vi "SetVIRef.vi"(8 "error in (no error)":errorcluster, 10 "VI Refnum":refnum<vi>, 11 "WindowFrame in":refnum<class "WindowFrame.lvclass">) -> (0 "error out":errorcluster, 3 "WindowFrame out":refnum<class "WindowFrame.lvclass">)   [LabVIEW 2021, in "WindowFrame.lvlib" / "WindowFrame.lvclass"]
uses:
  WindowFrame.lvclass
  C:/GitHub/ClassUtilities/src/ClassByRef/ClassByRef.lvclass
  ClassUtilities/src/ClassByRef/ClassByRef.lvclass/ClassByRef.ctl
  WindowFrame.lvclass/WindowFrame.ctl
  2388e8f5-2d87-4f60-8194-798a112a82ae.vi
  ClassUtilities/src/ClassByRef/GetRef.vi
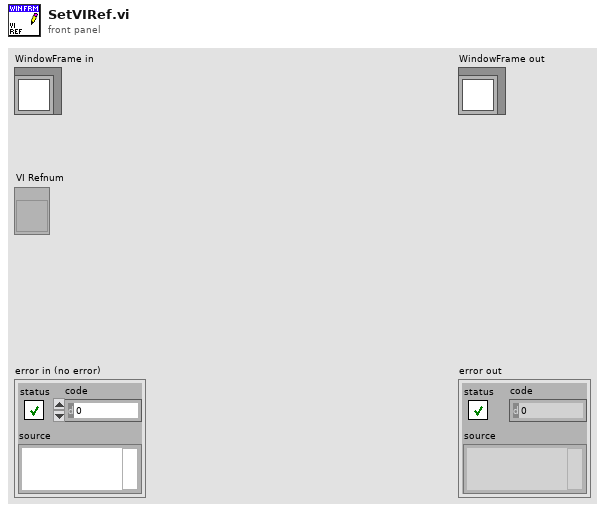
[diagram p1: front panel]
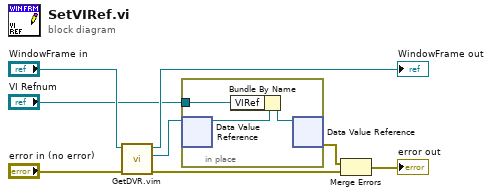
[diagram p0: block diagram]
diagram:
  n1 = call "GetDVR.vim"("error in (no error)"="error in (no error)", "ByRefClass in"="WindowFrame in") -> ("error out"=w1:errorcluster, "DVR"=w3:refnum<data-value>, "ByRefClass out"=→"WindowFrame out":refnum<class "WindowFrame.lvclass">)  [unwired: 7 in]
  n2 = in-place {
    in-place-border: "VI Refnum" -> [w10]
    n3 = in-place-dvr #1(w3) -> (w11:refnum<class "WindowFrame.lvclass">)  [unwired: 1 out]
    n4 = Bundle By Name(cluster=w11, "VIRef"=w10) -> (w9:refnum<class "WindowFrame.lvclass">)
    n5 = in-place-dvr #1(w9) -> (w2:errorcluster)  [unwired: 1 out]
  }
  n6 = Merge Errors(w2, w1) -> (→"error out":errorcluster)
